vi "GetText.vi"(8 "error in":errorcluster, 11 "OPC UA editor node in":refnum<class "OPC UA Client editor node.lvclass">) -> (0 "error out":errorcluster, 1 "additional text":string, 2 "text":string, 3 "OPC UA editor node out":refnum<class "OPC UA Client editor node.lvclass">, 4 "glyph":string)   [LabVIEW 2014, in "OPC UA Client editor node.lvclass"]
uses:
  OPC UA Client editor node.lvclass
  <vilib>/NI/DCAF/Tag Editor Core/Configuration Editor/Classes/Module editor node/Read display name.vi
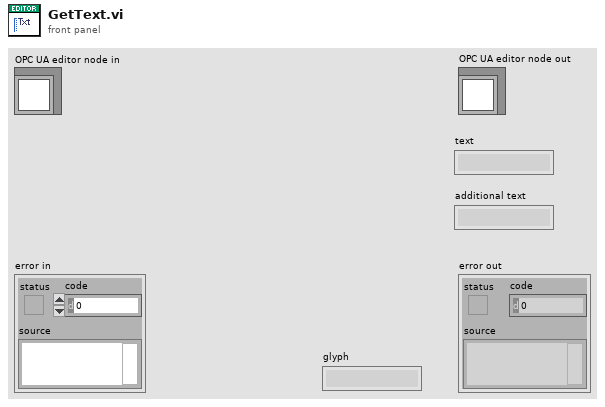
[diagram p1: front panel]
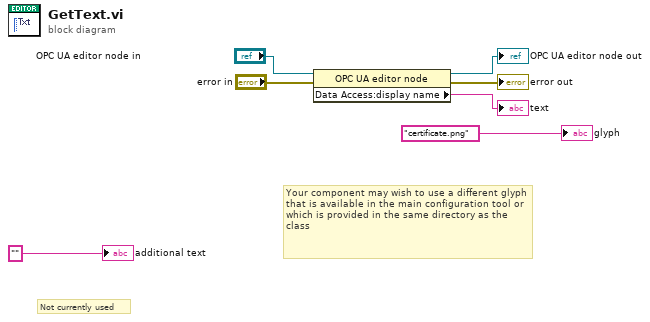
[diagram p0: block diagram]
diagram:
  # "Not currently used"
  # "Your component may wish to use a different glyph that is available in the main configuration tool or which is provided in the same directory as the class"
  n1 = property class="OPC UA editor node"(reference="OPC UA editor node in", error in="error in") -> (reference out=→"OPC UA editor node out":refnum<class "OPC UA Client editor node.lvclass">, error out=→"error out":errorcluster, "Data Access:display name"=→"text":string)
  "additional text" <- "" ("additional text")
  "glyph" <- "certificate.png" ("glyph")
